vi "AutoModEnable.vi"() -> ()   [LabVIEW 2016]
panel:
  out "Auto Mod Enable":bool
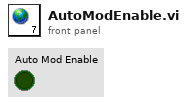
[diagram p1: front panel]
diagram:
